vi "Lift.vi"() -> ()   [LabVIEW 2018]
uses:
  <vilib>/Rock Robotics/SystemInterfaces/DIO/FPGA_DIOChannel.ctl
  <vilib>/Rock Robotics/WPI/ThirdParty/Phoenix-LabVIEW/Motor Controller/Controls/CTRE_Phoenix_MotorControl_ControlMode.ctl
  Times/Times Global.vi
  Lift Global.vi
  <vilib>/addons/control/pid/pid.llb/PID (DBL).vi
  <vilib>/Rock Robotics/WPI/ThirdParty/Phoenix-LabVIEW/Motor Controller/Get/CTRE_Phoenix_MotorController_GetSelectedSensorData.vi
  Cargo Intake/Cargo Intake Global.vi
  <vilib>/addons/control/pid/NI_PID_pid.lvlib
panel:
  in  "Output Scalar":dbl=1.0 format="%#_13g"
  in  "t":dbl=0.65 format="%#_13g"
  in  "output range":cluster{"output high":dbl, "output low":dbl}={"output high"=0.95, "output low"=-0.8}
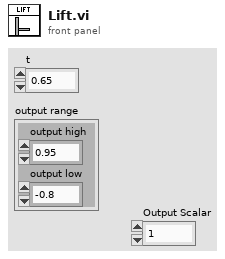
[diagram p1: front panel]
types:
  T1 = typedef "FPGA_DIOChannel.ctl" = enum8{"DIO 0", "DIO 1", "DIO 2", "DIO 3", "DIO 4", "DIO 5", "DIO 6", "DIO 7", "DIO 8", "DIO 9", "DIO MXP 0", "DIO MXP 1", "DIO MXP 2", "DIO MXP 3", "DIO MXP 4", "DIO MXP 5", "DIO MXP 6", "DIO MXP 7", "DIO MXP 8", "DIO MXP 9", "DIO MXP 10", "DIO MXP 11", "DIO MXP 12", "DIO MXP 13", "DIO MXP 14", "DIO MXP 15", "SPI Port CS1", "SPI Port CS2", "SPI Port CS3", "SPI Port MISO", "SPI Port MOSI", "Invalid"}
  T2 = typedef "WPI_MotorControlDeviceRef.ctl" = cluster{"DeviceStatus":errorcluster, "Type":T3, "PWM":cluster{"PWM Channel":T4, "DeadBand":T5}, "CAN":cluster{"Device Number":u8, "SetOutput VI Ref":variant, "GetOutput VI Ref":variant, "Enable VI Ref":variant, "Disable VI Ref":variant, "Data":variant}, "Invert":bool, "DIO PWM":cluster{"PWM \"Enable\" Channel":T4, "DIOChannel":T1, "PWM Rate":dbl}}
  T3 = typedef "WPI_MotorControlType.ctl" = enum16{"PWM", "CAN", "DIO PWM"}
  T4 = typedef "FPGA_DIOPWMChannel.ctl" = enum8{"PWM 0", "PWM 1", "PWM 2", "PWM 3", "PWM 4", "PWM 5", "PWM 6", "PWM 7", "PWM 8", "PWM 9", "PWM MXP 0", "PWM MXP 1", "PWM MXP 2", "PWM MXP 3", "PWM MXP 4", "PWM MXP 5", "PWM MXP 6", "PWM MXP 7", "PWM MXP 8", "PWM MXP 9", "Invalid"}
  T5 = typedef "WPI_PWMDeadband.ctl" = cluster{"Name":string, "maxPositivePwm":i32, "minPositivePwm":i32, "centerPwm":i32, "maxNegativePwm":i32, "minNegativePwm":i32, "angularRange":u16}
  T6 = typedef "WPI_DigitalInputDevRef.ctl" = cluster{"DevStatus":errorcluster, "DIO Channel":T1}
  T7 = typedef "CTRE_Phoenix_MotorControl_ControlMode.ctl" = u16
  T8 = cluster{"proportional gain (Kc)":dbl, "integral time(Ti, min)":dbl, "derivative time(Td, min) 2":dbl}
  T9 = enum16{"Hatch Panel Zone 1", "Hatch Panel Zone 2", "Hatch Panel Zone 3", "Cargo Zone 1", "Cargo Zone 2", "Cargo Zone 3", "Cargo Ship Zone"}
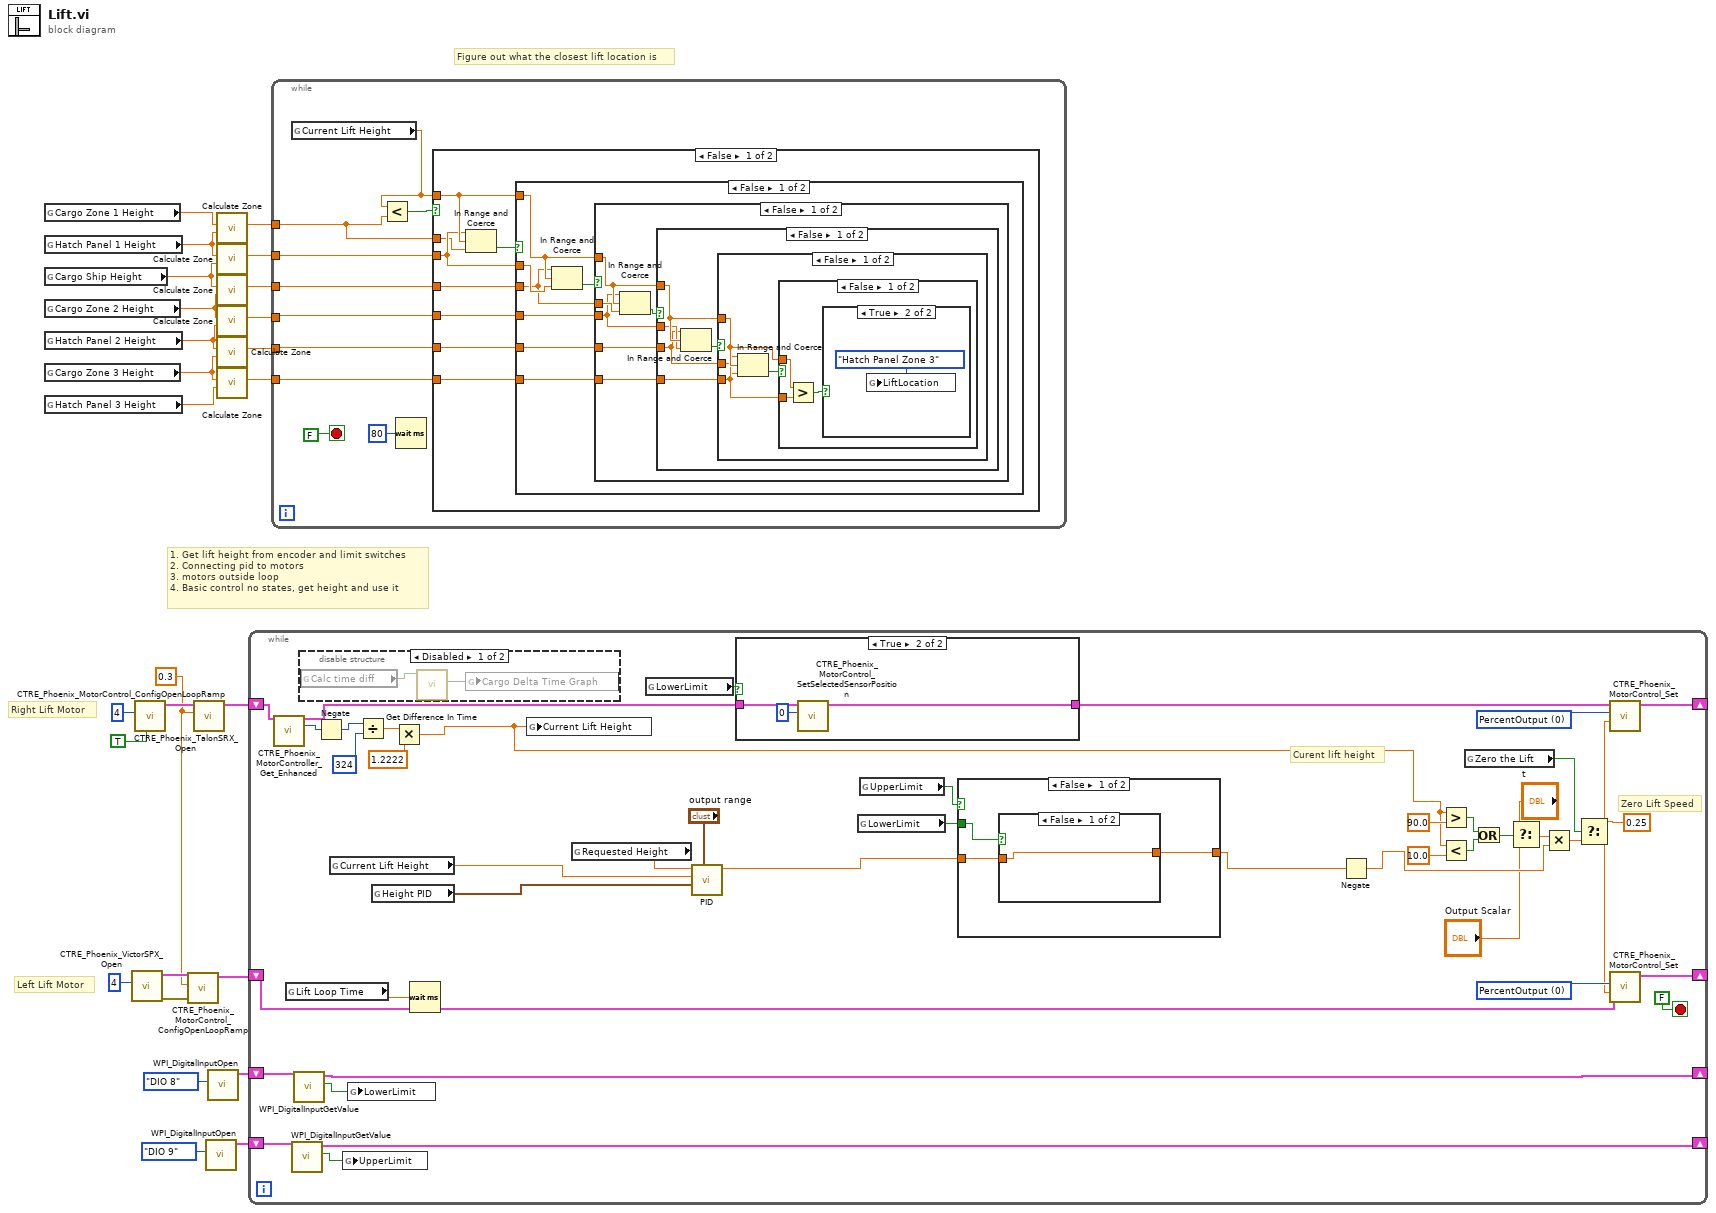
[diagram p0: block diagram]
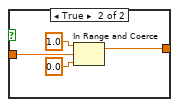
[diagram p2: hidden frame]
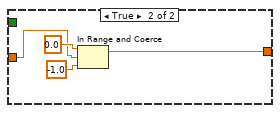
[diagram p3: hidden frame]
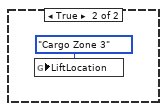
[diagram p7: hidden frame]
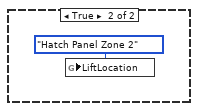
[diagram p8: hidden frame]
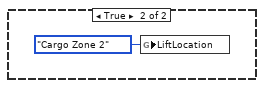
[diagram p9: hidden frame]
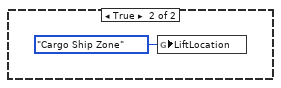
[diagram p10: hidden frame]
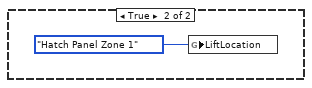
[diagram p11: hidden frame]
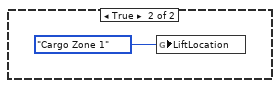
[diagram p12: hidden frame]
diagram:
  w2 = 0.3 ("secondsFromNeutralToFull")
  # "Left Lift Motor"
  # "Right Lift Motor"
  # "Figure out what the closest lift location is"
  # "1. Get lift height from encoder and limit switches\n2. Connecting pid to motors\n3. motors outside loop\n4. Basic control no states, get height and use it"
  n1 = global read "Lift Global.vi" "Cargo Zone 1 Height"() -> (w20:dbl)
  n2 = global read "Lift Global.vi" "Hatch Panel 1 Height"() -> (w26:dbl)
  n3 = global read "Lift Global.vi" "Cargo Ship Height"() -> (w25:dbl)
  n4 = global read "Lift Global.vi" "Cargo Zone 2 Height"() -> (w24:dbl)
  n5 = global read "Lift Global.vi" "Hatch Panel 2 Height"() -> (w23:dbl)
  n6 = global read "Lift Global.vi" "Cargo Zone 3 Height"() -> (w22:dbl)
  n7 = global read "Lift Global.vi" "Hatch Panel 3 Height"() -> (w21:dbl)
  n8 = call <vilib>:"CTRE_Phoenix_VictorSPX_Open.vi"("Device Number"=u8 4) -> ("error out"=w5:errorcluster, "CAN Talon SRX Ref"=w4:T2)  [unwired: 9 in]
  n9 = call <vilib>:"CTRE_Phoenix_TalonSRX_Open.vi"("Invert"=TRUE, "Device Number"=u8 4) -> ("CAN Talon SRX Ref"=w7:T2)  [unwired: 8 in, 1 out]
  n10 = call <vilib>:"CTRE_Phoenix_MotorControl_ConfigOpenLoopRamp.vi"("error in (no error)"=w5, "secondsFromNeutralToFull"=w2, "PhoenixMotorControlDevRef"=w4) -> ("PhoenixMotorControlDevRef"=w3:T2)  [unwired: 7 in, 1 out]
  n11 = call <vilib>:"CTRE_Phoenix_MotorControl_ConfigOpenLoopRamp.vi"("secondsFromNeutralToFull"=w2, "PhoenixMotorControlDevRef"=w7) -> ("PhoenixMotorControlDevRef"=w6:T2)  [unwired: 8 in, 1 out]
  n12 = call <vilib>:"WPI_DigitalInputOpen.vi"("DIO Channel"=FPGA_DIOChannel."DIO 9") -> ("DigitalInputDevRef"=w8:T6)  [unwired: 9 in, 1 out]
  n13 = call <vilib>:"WPI_DigitalInputOpen.vi"("DIO Channel"=FPGA_DIOChannel."DIO 8") -> ("DigitalInputDevRef"=w10:T6)  [unwired: 9 in, 1 out]
  n14 = call "Calculate Zone.vi"("Top Height"=w26, "Bottom Height"=w20) -> ("Midpoint"=w19:dbl)  [unwired: 9 in]
  n15 = call "Calculate Zone.vi"("Top Height"=w25, "Bottom Height"=w26) -> ("Midpoint"=w18:dbl)  [unwired: 9 in]
  n16 = call "Calculate Zone.vi"("Top Height"=w24, "Bottom Height"=w25) -> ("Midpoint"=w17:dbl)  [unwired: 9 in]
  n17 = call "Calculate Zone.vi"("Top Height"=w23, "Bottom Height"=w24) -> ("Midpoint"=w16:dbl)  [unwired: 9 in]
  n18 = call "Calculate Zone.vi"("Top Height"=w22, "Bottom Height"=w23) -> ("Midpoint"=w15:dbl)  [unwired: 9 in]
  n19 = call "Calculate Zone.vi"("Top Height"=w21, "Bottom Height"=w22) -> ("Midpoint"=w14:dbl)  [unwired: 9 in]
  n20 = while {
    shift-right: [w67] -> _
    shift-left: w6 -> [w60]
    shift-right: [w65] -> _
    shift-left: w3 -> [w64]
    shift-right: [w55] -> _
    shift-left: w10 -> [w56]
    shift-right: [w50] -> _
    shift-left: w8 -> [w51]
    stop <- FALSE stop-if-true
    w66 = T7 0 items=["PercentOutput"=0, "Position"=1, "Velocity"=2, "Current"=3, "Follower"=5, "MotionProfile"=6, "MotionMagic"=7, "MotionProfileArc"=10, "Disabled"=15] ("Control Mode")
    w68 = T7 0 items=["PercentOutput"=0, "Position"=1, "Velocity"=2, "Current"=3, "Follower"=5, "MotionProfile"=6, "MotionMagic"=7, "MotionProfileArc"=10, "Disabled"=15] ("Control Mode")
    # "Curent lift height"
    # "Zero Lift Speed"
    n21 = call-poly <vilib>:"CTRE_Phoenix_MotorController_Get_Enhanced.vi"("PhoenixMotorControlDevRef"=w60) -> ("PhoenixMotorControlDevRef"=w59:T2, "Position (Raw Sensor Units)"=w33:i32)  [unwired: 11 in, 2 out]
    n22 = global read "Times Global.vi" "Lift Loop Time"() -> (w70:dbl)
    n23 = call <vilib>:"WPI_DigitalInputGetValue.vi"("DigitalInputDevRef"=w51) -> ("Value"=w53:bool, "DigitalInputDevRef"=w50:T6)  [unwired: 8 in, 1 out]
    n24 = call <vilib>:"WPI_DigitalInputGetValue.vi"("DigitalInputDevRef"=w56) -> ("Value"=w54:bool, "DigitalInputDevRef"=w55:T6)  [unwired: 8 in, 1 out]
    n25 = disable-structure shown="Disabled" {
      frame Disabled {
        n26 = global read "Cargo Intake Global.vi" "Calc time diff"() -> (w88:bool)
        n27 = call "Get Difference In Time.vi"("Calculate Time Difference"=w88) -> ("Delta Time over Time"=w87:u32)  [unwired: 9 in, 1 out]
        n28 = global write "Times Global.vi" "Cargo Delta Time Graph"(w87) -> ()
      }
      frame Enabled {
      }
    }
    n29 = Negate(x=w33) -> (-x=w34:i32)
    n30 = global read "Lift Global.vi" "Current Lift Height"() -> (w61:dbl)
    n31 = global write "Lift Global.vi" "UpperLimit"(w53) -> ()
    n32 = global write "Lift Global.vi" "LowerLimit"(w54) -> ()
    n33 = Divide(x=w34, y=324) -> (x/y=w40:dbl)
    n34 = global read "Lift Global.vi" "Height PID"() -> (w62:T8)
    n35 = Multiply(x=w40, y=1.2222) -> (x*y=w27:dbl)
    n36 = Wait (ms)(milliseconds to wait=w70) -> ()  [unwired: 1 out]
    n37 = global write "Lift Global.vi" "Current Lift Height"(w27) -> ()
    n38 = global read "Lift Global.vi" "Requested Height"() -> (w28:dbl)
    n39 = global read "Lift Global.vi" "LowerLimit"() -> (w52:bool)
    n40 = call-poly <vilib>:"PID.vi"("output range"="output range", "PID gains"=w62, "process variable"=w61, "setpoint"=w28) -> ("output"=w30:dbl)  [unwired: 6 in, 1 out]
    n41 = case shown="True" w52 {
      tunnel: w59 -> [w83 w86]
      tunnel: [w83 w85] -> w58
      frame False {
      }
      frame True {
        n42 = call <vilib>:"CTRE_Phoenix_MotorControl_SetSelectedSensorPosition.vi"("New Sensor Position"=0, "PhoenixMotorControlDevRef"=w86) -> ("PhoenixMotorControlDevRef"=w85:T2)  [unwired: 8 in, 1 out]
      }
    }
    n43 = global read "Lift Global.vi" "LowerLimit"() -> (w32:bool)
    n44 = global read "Lift Global.vi" "UpperLimit"() -> (w31:bool)
    n45 = case shown="False" w31 {
      tunnel: w32 -> [w73 _]
      tunnel: [w72 w80] -> w29
      tunnel: w30 -> [w71 w79]
      frame False {
        n46 = case shown="False" w73 {
          tunnel: [w74 w78] -> w72
          tunnel: w71 -> [w74 w75]
          frame False {
          }
          frame True {
            n47 = In Range and Coerce(upper limit=1.0, x=w75, lower limit=0.0) -> (coerced(x)=w78:dbl)  [unwired: 1 out]
          }
        }
      }
      frame True {
        n48 = In Range and Coerce(upper limit=0.0, x=w79, lower limit=-1.0) -> (coerced(x)=w80:dbl)  [unwired: 1 out]
      }
    }
    n49 = Negate(x=w29) -> (-x=w43:dbl)
    n50 = Greater?(x=w27, y=90.0) -> (0:w46:bool)
    n51 = Less?(x=w27, y=10.0) -> (x < y?=w47:bool)
    n52 = global read "Lift Global.vi" "Zero the Lift"() -> (w37:bool)
    n53 = Or(x=w46, y=w47) -> (x .or. y?=w45:bool)
    n54 = Select(t="t", s=w45, f="Output Scalar") -> (s? t:f=w44:dbl)
    n55 = Multiply(x=w44, y=w43) -> (x*y=w38:dbl)
    n56 = Select(t=0.25, s=w37, f=w38) -> (s? t:f=w35:dbl)
    n57 = call <vilib>:"CTRE_Phoenix_MotorControl_Set.vi"("Output"=w35, "Control Mode"=w68, "PhoenixMotorControlDevRef"=w58) -> ("PhoenixMotorControlDevRef"=w67:T2)  [unwired: 7 in, 1 out]
    n58 = call <vilib>:"CTRE_Phoenix_MotorControl_Set.vi"("Output"=w35, "Control Mode"=w66, "PhoenixMotorControlDevRef"=w64) -> ("PhoenixMotorControlDevRef"=w65:T2)  [unwired: 7 in, 1 out]
  }
  n59 = while {
    tunnel: w19 -> [w94]
    tunnel: w18 -> [w93]
    tunnel: w17 -> [w92]
    tunnel: w16 -> [w91]
    tunnel: w15 -> [w90]
    tunnel: w14 -> [w89]
    stop <- FALSE stop-if-true
    n60 = global read "Lift Global.vi" "Current Lift Height"() -> (w95:dbl)
    n61 = Less?(x=w95, y=w94) -> (x < y?=w96:bool)
    n62 = Wait (ms)(milliseconds to wait=u32 80) -> ()  [unwired: 1 out]
    n63 = case shown="False" w96 {
      tunnel: w95 -> [w102 _]
      tunnel: w94 -> [w100 _]
      tunnel: w93 -> [w101 _]
      tunnel: w92 -> [w106 _]
      tunnel: w91 -> [w105 _]
      tunnel: w90 -> [w104 _]
      tunnel: w89 -> [w103 _]
      frame False {
        n64 = In Range and Coerce(upper limit=w101, x=w102, lower limit=w100) -> (In Range?=w99:bool)  [unwired: 1 out]
        n65 = case shown="False" w99 {
          tunnel: w102 -> [w109 _]
          tunnel: w101 -> [w108 _]
          tunnel: w106 -> [w107 _]
          tunnel: w105 -> [w113 _]
          tunnel: w104 -> [w112 _]
          tunnel: w103 -> [w111 _]
          frame False {
            n66 = In Range and Coerce(upper limit=w107, x=w109, lower limit=w108) -> (In Range?=w110:bool)  [unwired: 1 out]
            n67 = case shown="False" w110 {
              tunnel: w109 -> [w116 _]
              tunnel: w113 -> [w114 _]
              tunnel: w112 -> [w119 _]
              tunnel: w111 -> [w118 _]
              tunnel: w107 -> [w115 _]
              frame False {
                n68 = In Range and Coerce(upper limit=w114, x=w116, lower limit=w115) -> (In Range?=w117:bool)  [unwired: 1 out]
                n69 = case shown="False" w117 {
                  tunnel: w116 -> [w122 _]
                  tunnel: w119 -> [w120 _]
                  tunnel: w118 -> [w124 _]
                  tunnel: w114 -> [w121 _]
                  frame False {
                    n70 = In Range and Coerce(upper limit=w120, x=w122, lower limit=w121) -> (In Range?=w123:bool)  [unwired: 1 out]
                    n71 = case shown="False" w123 {
                      tunnel: w122 -> [w127 _]
                      tunnel: w124 -> [w126 _]
                      tunnel: w120 -> [w125 _]
                      frame False {
                        n72 = In Range and Coerce(upper limit=w126, x=w127, lower limit=w125) -> (In Range?=w128:bool)  [unwired: 1 out]
                        n73 = case shown="False" w128 {
                          tunnel: w127 -> [w131 _]
                          tunnel: w126 -> [w130 _]
                          frame False {
                            n74 = Greater?(x=w131, y=w130) -> (0:w129:bool)
                            n75 = case shown="True" w129 {
                              frame False {
                              }
                              frame True {
                                n76 = global write "Lift Global.vi" "LiftLocation"(T9."Hatch Panel Zone 3" ("LiftLocation")) -> ()
                              }
                            }
                          }
                          frame True {
                            n77 = global write "Lift Global.vi" "LiftLocation"(T9."Cargo Zone 3" ("LiftLocation")) -> ()
                          }
                        }
                      }
                      frame True {
                        n78 = global write "Lift Global.vi" "LiftLocation"(T9."Hatch Panel Zone 2" ("LiftLocation")) -> ()
                      }
                    }
                  }
                  frame True {
                    n79 = global write "Lift Global.vi" "LiftLocation"(T9."Cargo Zone 2" ("LiftLocation")) -> ()
                  }
                }
              }
              frame True {
                n80 = global write "Lift Global.vi" "LiftLocation"(T9."Cargo Ship Zone" ("LiftLocation")) -> ()
              }
            }
          }
          frame True {
            n81 = global write "Lift Global.vi" "LiftLocation"(T9."Hatch Panel Zone 1" ("LiftLocation")) -> ()
          }
        }
      }
      frame True {
        n82 = global write "Lift Global.vi" "LiftLocation"(T9."Cargo Zone 1" ("LiftLocation")) -> ()
      }
    }
  }
